vi "OCV DAQ Software Trigger.vi"(8 "error in (no error)":errorcluster, 10 "Timeout (ms)":u32=30000, 11 "Refnum in":refnum<k21>) -> (0 "error out":errorcluster, 3 "Refnum out":refnum<k21>, 4 "Trigger Time (ms)":u32=19055974)   [LabVIEW 2019]
panel:
  out "millisecond timer value out":u32=19055976
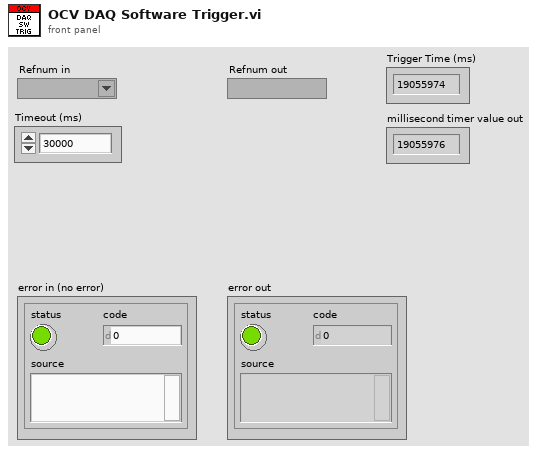
[diagram p1: front panel]
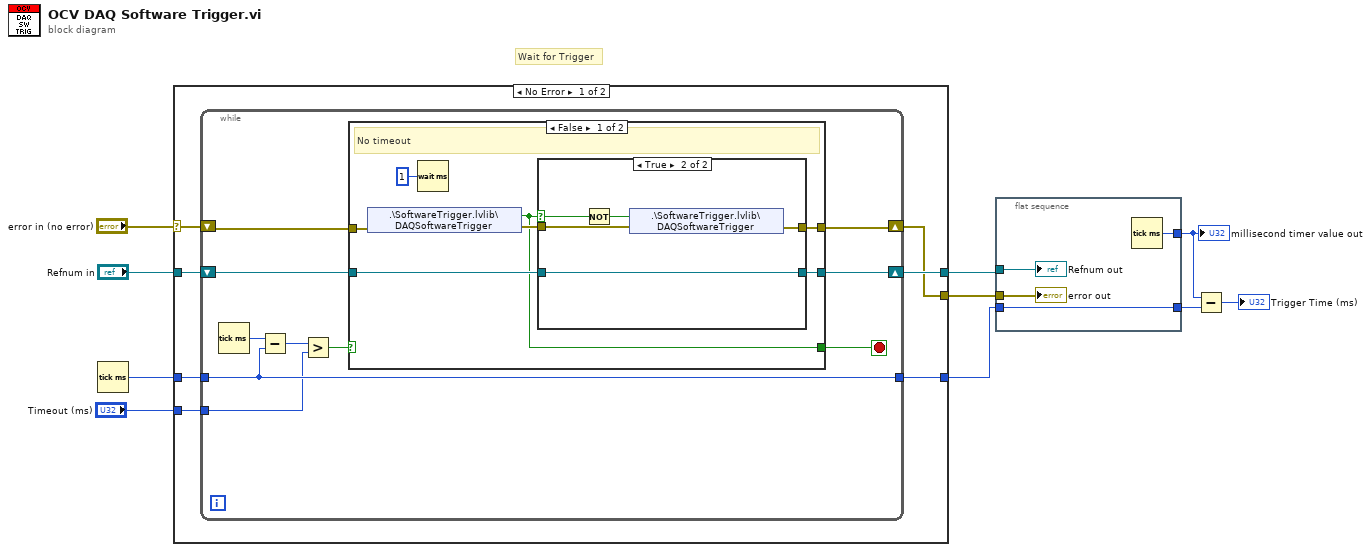
[diagram p0: block diagram]
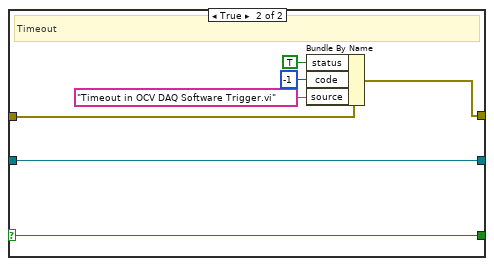
[diagram p3: hidden frame]
diagram:
  # "Wait for Trigger"
  n1 = Tick Count (ms)() -> (millisecond timer value=w4:u32)
  n2 = case shown="No Error" "error in (no error)" {
    selector: "error in (no error)" -> [w11 w51]
    tunnel: "Refnum in" -> [w17 w50]
    tunnel: [w16 w50] -> w6
    tunnel: [w15 w51] -> w5
    tunnel: w4 -> [w14 w49]
    tunnel: [w13 w49] -> w3
    tunnel: "Timeout (ms)" -> [w12 _]
    frame No Error {
      n3 = while {
        shift-right: [w26] -> w15
        shift-left: w11 -> [w27]
        shift-right: [w24] -> w16
        shift-left: w17 -> [w25]
        tunnel: w14 -> [w22]
        tunnel: [w22] -> w13
        tunnel: w12 -> [w20]
        stop <- w18 stop-if-true
        n4 = Tick Count (ms)() -> (millisecond timer value=w23:u32)
        n5 = Subtract(x=w23, y=w22) -> (x-y=w21:u32)
        n6 = Greater?(x=w21, y=w20) -> (0:w19:bool)
        n7 = case shown="False" w19 {
          selector: w19 -> [_ w47]
          tunnel: w27 -> [w33 w46]
          tunnel: [w31 w45] -> w26
          tunnel: w25 -> [w30 w48]
          tunnel: [w29 w48] -> w24
          tunnel: [w28 w47] -> w18
          frame False {
            # "No timeout"
            n8 = shared-variable ".\\SoftwareTrigger.lvlib\\DAQSoftwareTrigger"(error in=w33) -> (w28:bool, error out=w32:errorcluster)
            n9 = Wait (ms)(milliseconds to wait=u32 1) -> ()  [unwired: 1 out]
            n10 = case shown="True" w28 {
              selector: w28 -> [_ w39]
              tunnel: w32 -> [w36 w41]
              tunnel: [w36 w40] -> w31
              tunnel: w30 -> [w35 w37]
              tunnel: [w35 w37] -> w29
              frame False {
              }
              frame True {
                n11 = Not(x=w39) -> (.not. x?=w38:bool)
                n12 = shared-variable ".\\SoftwareTrigger.lvlib\\DAQSoftwareTrigger"(w38, error in=w41) -> (error out=w40:errorcluster)
              }
            }
          }
          frame True {
            # "Timeout"
            n13 = Bundle By Name(cluster=w46, "status"=TRUE, "code"=-1, "source"="Timeout in OCV DAQ Software Trigger.vi") -> (w45:errorcluster)
          }
        }
      }
    }
    frame Error {
    }
  }
  n14 = flat-sequence {
    tunnel: [w55] -> w8
    tunnel: w3 -> [w54]
    tunnel: [w54] -> w9
    tunnel: w6 -> [w53]
    tunnel: w5 -> [w52]
    frame #0 {
      n15 = Tick Count (ms)() -> (millisecond timer value=w55:u32)
      "Refnum out" <- w53
      "error out" <- w52
    }
  }
  n16 = Subtract(x=w8, y=w9) -> (x-y=→"Trigger Time (ms)":u32)
  "millisecond timer value out" <- w8
